vi "Get Speaker State.vi"(8 "error in":errorcluster, 11 "PAS in":refnum<class "PAS.lvclass">) -> (0 "error out":errorcluster, 2 "State":bool, 3 "PAS out":refnum<class "PAS.lvclass">)   [LabVIEW 2014, in "PAS Library.lvlib" / "PAS.lvclass"]
uses:
  PAS.lvclass
  PAS.lvclass/PAS.ctl
  Switch/Switch.lvclass
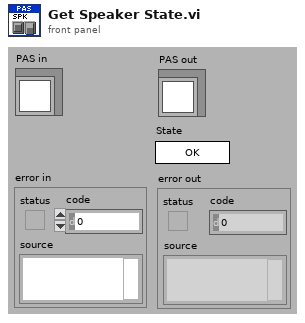
[diagram p1: front panel]
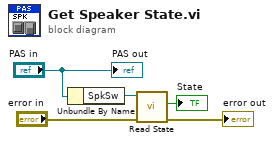
[diagram p0: block diagram]
diagram:
  n1 = Unbundle By Name("PAS in") -> ("SpkSw"=w2:refnum<class "Switch.lvclass">)
  n2 = call-dynamic "Read State.vi"("error in (no error)"="error in", "Switch in"=w2) -> ("error out"=→"error out":errorcluster, "State"=→"State":bool)  [unwired: 7 in, 1 out]
  "PAS out" <- "PAS in"
